vi "Overshoot Function (SubVI).vi"(0 "Signals IN":T2={"Dispense"=FALSE, "Fill"=FALSE, "Spray"=FALSE, "Drain"=TRUE, "Complete"=FALSE, "Fill Error"=FALSE, "Dispense Error"=FALSE, "Fill Timeout"=FALSE, "Dispense Timeout"=FALSE}, 1 "Values IN":T3 {"Drain Time (s)" format="%.2f"; "Drain Rate (g/sec)" format="%.2f"; "Time Elapsed (s)" format="%.2f"; "Time Target (s)" format="%.2f"; "Dynamic Setpoint (g)" format="%.2f"; "Static Setpoint (g)" format="%.2f"; "Grams to Setpoint" format="%.2f"; "Adjusted Mass (g)" format="%.2f"; "Dispense Rate (g/sec)" format="%.2f"; "Fill Mass (g)" format="%.2f"; "Fill Rate (g/sec)" format="%.2f"}, 3 "Settings":T1={"ON Settings"={"Enable Dynamic Setpoint?"=TRUE, "Enable Dynamic Dispense Time?"=TRUE, "Enable Drain Rate Functions"=TRUE, "Dispense Sample Time (s)"=0.5, "Dispense Slope Ave"=0, "ON Timeout (sec)"=600.0, "1st Setpoint (% of Target)"=0.0, "2nd Setpoint (% of Target)"=0.0, "3rd Setpoint (% of Target)"=0.0, "Measure Dispense Delay (sec)"=0.0, "Settle Slope Sample Time (s)"=0.0}, "OFF Settings"={"Drain Sample Time (s)"=0.5, "Drain Rate Ave Size"=5, "Drain Rate Limits (± g/sec)"=10.0, "Level Slope Range (± g/sec)"=0.25, "OFF Timeout (sec)"=0.0, "Near SP Slope Level (± g/sec)"=0.01, "Near Setpoint Threshold (%)"=95.0}, "Overshoot Settings"={"Time Limit (s)"=60.0, "Container MAX (g)"=1500.0, "Max FILL Slope (+/- g/sec)"=10.0, "% Overshot to Enable (>)"=0.25}, "FILL Timeout (s)"=300.0, "Full Settle Time (s)"=3.0, "Pre-Hydrate \nSpray Time (s)"=10.0, "Pre-Hydrate \nWait Time (s)"=30.0}, 5 "Measured Mass (g)":dbl) -> (14 "Signals OUT":T2={"Dispense"=FALSE, "Fill"=FALSE, "Spray"=FALSE, "Drain"=TRUE, "Complete"=FALSE, "Fill Error"=FALSE, "Dispense Error"=FALSE, "Fill Timeout"=FALSE, "Dispense Timeout"=FALSE}, 15 "Values OUT":T3 {"Drain Time (s)" format="%.2f"; "Drain Rate (g/sec)" format="%.2f"; "Time Elapsed (s)" format="%.2f"; "Time Target (s)" format="%.2f"; "Dynamic Setpoint (g)" format="%.2f"; "Static Setpoint (g)" format="%.2f"; "Grams to Setpoint" format="%.2f"; "Adjusted Mass (g)" format="%.2f"; "Dispense Rate (g/sec)" format="%.2f"; "Fill Mass (g)" format="%.2f"; "Fill Rate (g/sec)" format="%.2f"}, 17 "Fill Target (g)":dbl, 18 "Fill Time Target (s)":dbl, 19 "Complete":bool)   [LabVIEW 2009]
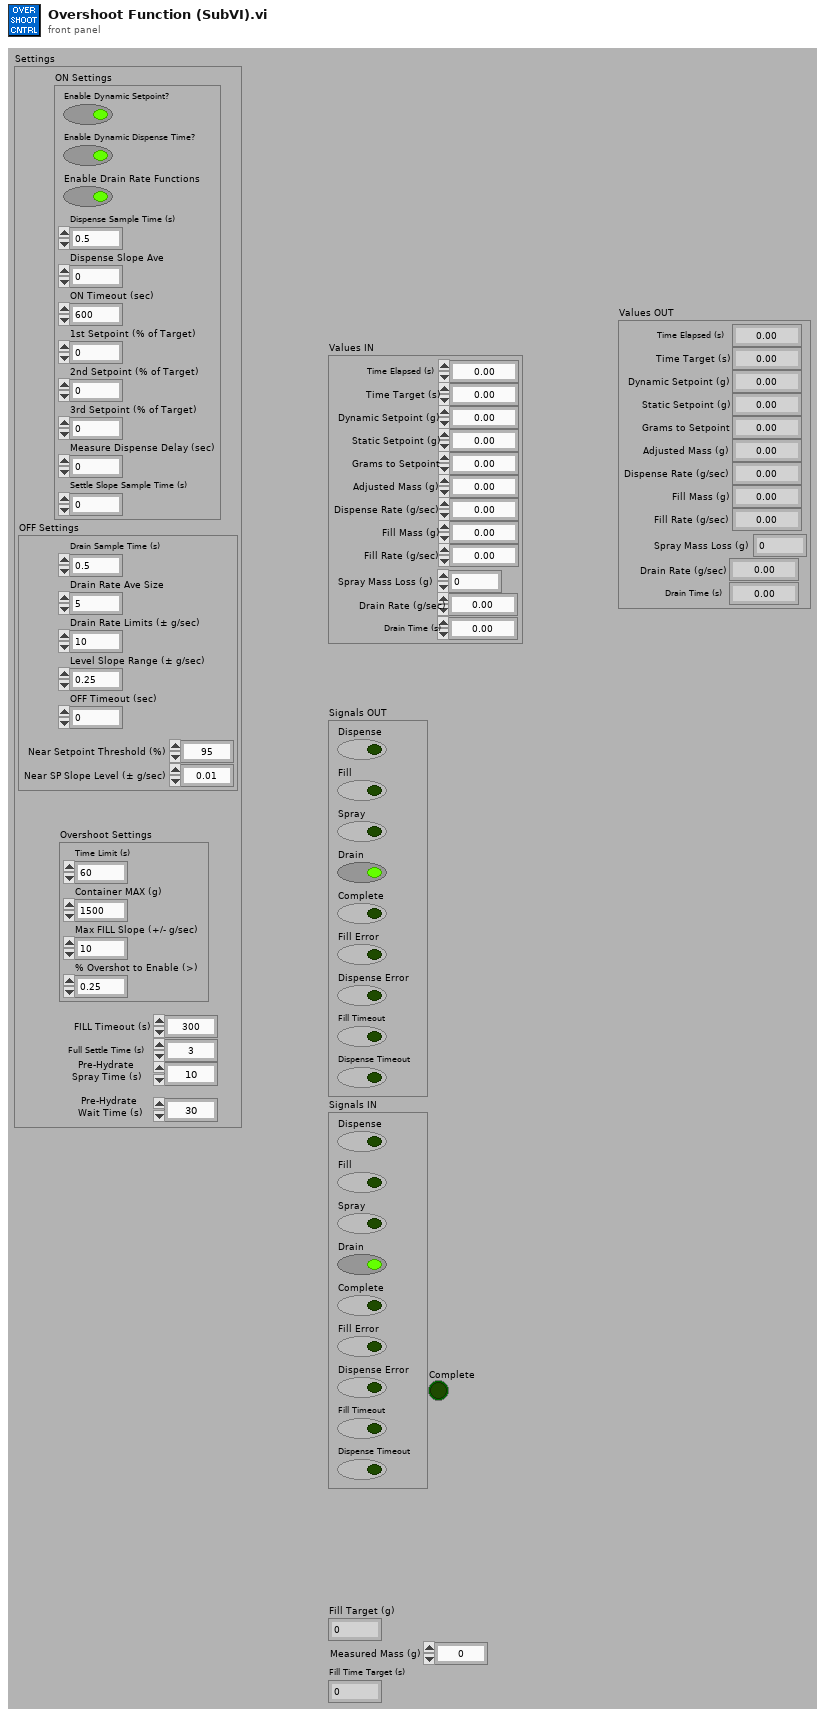
[diagram p1: front panel]
types:
  T1 = cluster{"ON Settings":cluster{"Enable Dynamic Setpoint?":bool, "Enable Dynamic Dispense Time?":bool, "Enable Drain Rate Functions":bool, "Dispense Sample Time (s)":dbl, "Dispense Slope Ave":i32, "ON Timeout (sec)":dbl, "1st Setpoint (% of Target)":dbl, "2nd Setpoint (% of Target)":dbl, "3rd Setpoint (% of Target)":dbl, "Measure Dispense Delay (sec)":dbl, "Settle Slope Sample Time (s)":dbl}, "OFF Settings":cluster{"Drain Sample Time (s)":dbl, "Drain Rate Ave Size":i32, "Drain Rate Limits (± g/sec)":dbl, "Level Slope Range (± g/sec)":dbl, "OFF Timeout (sec)":dbl, "Near SP Slope Level (± g/sec)":dbl, "Near Setpoint Threshold (%)":dbl}, "Overshoot Settings":cluster{"Time Limit (s)":dbl, "Container MAX (g)":dbl, "Max FILL Slope (+/- g/sec)":dbl, "% Overshot to Enable (>)":dbl}, "FILL Timeout (s)":dbl, "Full Settle Time (s)":dbl, "Pre-Hydrate \nSpray Time (s)":dbl, "Pre-Hydrate \nWait Time (s)":dbl}
  T2 = cluster{"Dispense":bool, "Fill":bool, "Spray":bool, "Drain":bool, "Complete":bool, "Fill Error":bool, "Dispense Error":bool, "Fill Timeout":bool, "Dispense Timeout":bool}
  T3 = cluster{"Time Elapsed (s)":dbl, "Time Target (s)":dbl, "Dynamic Setpoint (g)":dbl, "Static Setpoint (g)":dbl, "Grams to Setpoint":dbl, "Adjusted Mass (g)":dbl, "Dispense Rate (g/sec)":dbl, "Fill Mass (g)":dbl, "Fill Rate (g/sec)":dbl, "Spray Mass Loss (g)":dbl, "Drain Rate (g/sec)":dbl, "Drain Time (s)":dbl}
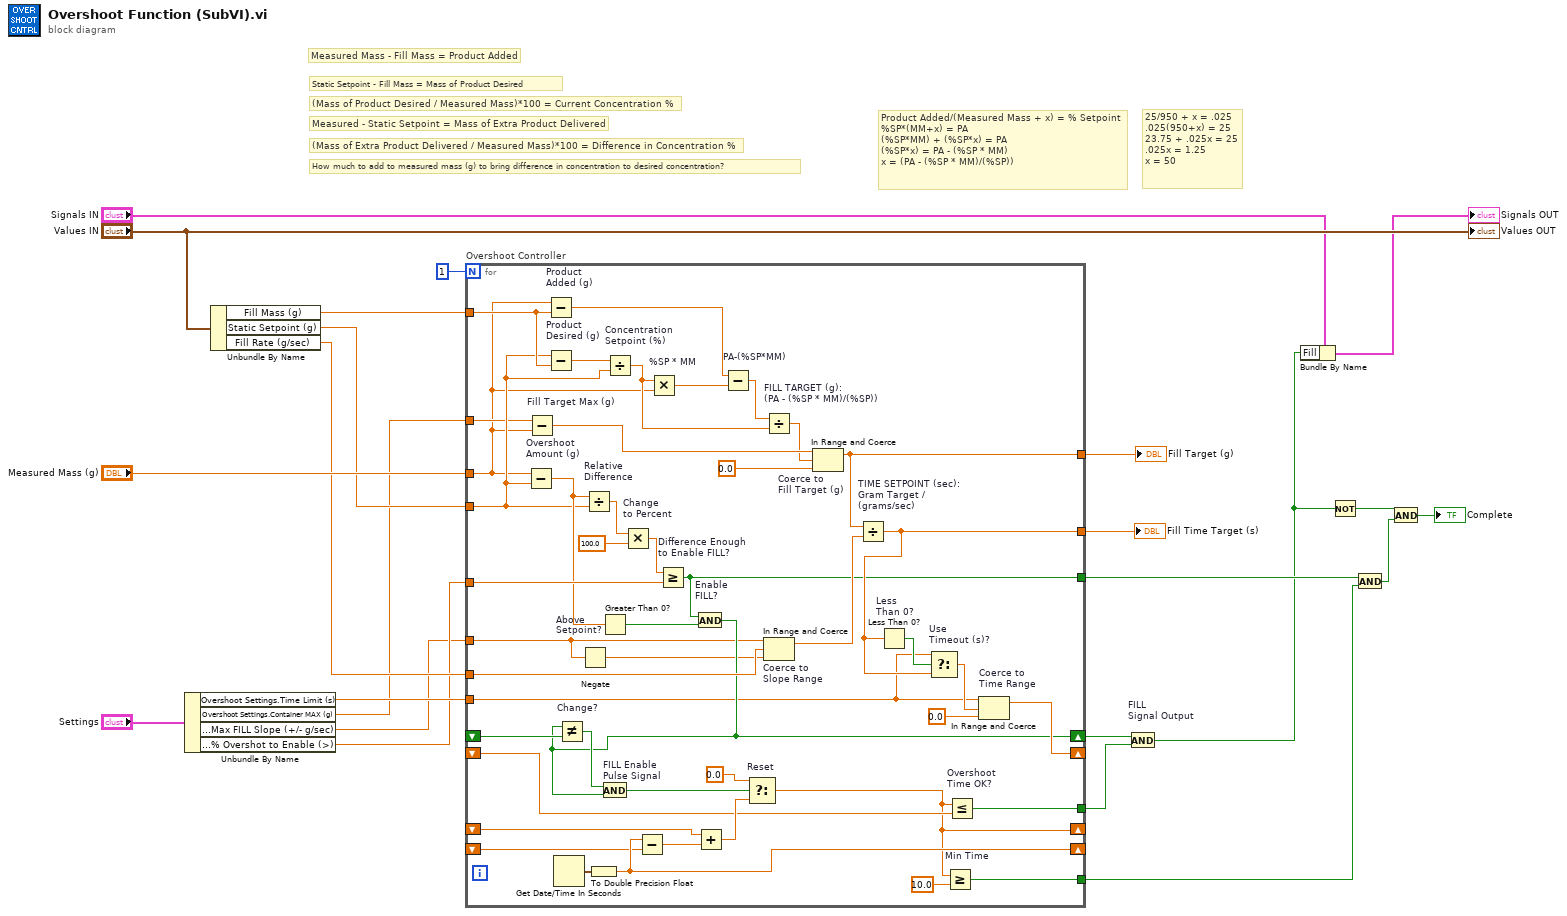
[diagram p0: block diagram]
diagram:
  # "Measured Mass - Fill Mass = Product Added"
  # "Product Added/(Measured Mass + x) = % Setpoint\n%SP*(MM+x) = PA\n(%SP*MM) + (%SP*x) = PA\n(%SP*x) = PA - (%SP * MM)\nx = (PA - (%SP * MM)/(%SP))"
  # "25/950 + x = .025\n.025(950+x) = 25\n23.75 + .025x = 25\n.025x = 1.25\nx = 50"
  # "How much to add to measured mass (g) to bring difference in concentration to desired concentration?"
  # "(Mass of Extra Product Delivered / Measured Mass)*100 = Difference in Concentration %"
  # "(Mass of Product Desired / Measured Mass)*100 = Current Concentration %"
  # "Measured - Static Setpoint = Mass of Extra Product Delivered"
  # "Static Setpoint - Fill Mass = Mass of Product Desired"
  n1 = Unbundle By Name("Settings") -> ("Overshoot Settings.Time Limit (s)"=w4:dbl, "Overshoot Settings.Container MAX (g)"=w2:dbl, "Overshoot Settings.Max FILL Slope (+/- g/sec)"=w1:dbl, "Overshoot Settings.% Overshot to Enable (>)"=w3:dbl)
  n2 = Unbundle By Name("Values IN") -> ("Fill Mass (g)"=w15:dbl, "Static Setpoint (g)"=w16:dbl, "Fill Rate (g/sec)"=w17:dbl)
  n3 = for "Overshoot Controller" {
    N: 1 -> [_]
    shift-right: [w26] -> _
    shift-left: _ -> [w69]
    shift-right: [w65] -> _
    shift-left: _ -> [w64]
    tunnel: [w66] -> w19
    shift-right: [w31] -> w20
    shift-left: _ -> [w62]
    shift-right: [w59] -> _
    shift-left: _ -> [w58]
    tunnel: w1 -> [w30]
    tunnel: w17 -> [w48]
    tunnel: w3 -> [w47]
    tunnel: w16 -> [w43]
    tunnel: "Measured Mass (g)" -> [w36]
    tunnel: w15 -> [w45]
    tunnel: [w33] -> w22
    tunnel: w2 -> [w37]
    tunnel: [w32] -> w23
    tunnel: w4 -> [w28]
    tunnel: [w27] -> w11
    tunnel: [w24] -> w10
    n4 = Subtract "Overshoot\nAmount (g)"(x=w36, y=w43) -> (x-y=w46:dbl)
    n5 = Subtract "Fill Target Max (g)"(x=w37, y=w36) -> (x-y=w35:dbl)
    n6 = Subtract "Product\nAdded (g)"(x=w36, y=w45) -> (x-y=w42:dbl)
    n7 = Subtract "Product\nDesired (g)"(x=w43, y=w45) -> (x-y=w44:dbl)
    n8 = Get Date/Time In Seconds() -> (seconds since 1Jan1904=w68:timestamp)
    n9 = Negate(x=w30) -> (-x=w29:dbl)
    n10 = Divide "Relative\nDifference"(x=w46, y=w43) -> (x/y=w50:dbl)
    n11 = To Double Precision Float(number=w68) -> (double precision float=w65:dbl)
    n12 = Greater Than 0? "Above\nSetpoint?"(x=w46) -> (x > 0?=w49:bool)
    n13 = Divide "Concentration\nSetpoint (%)"(x=w44, y=w43) -> (x/y=w39:dbl)
    n14 = Multiply "Change\nto Percent"(x=w50, y=100.0) -> (x*y=w52:dbl)
    n15 = Subtract(x=w65, y=w64) -> (x-y=w63:dbl)
    n16 = Multiply "%SP * MM"(x=w39, y=w36) -> (x*y=w41:dbl)
    n17 = Greater Or Equal? "Difference Enough\nto Enable FILL?"(x=w52, y=w47) -> (x >= y?=w27:bool)
    n18 = And "Enable\nFILL?"(x=w27, y=w49) -> (x .and. y?=w31:bool)
    n19 = Not Equal? "Change?"(x=w31, y=w62) -> (x != y?=w61:bool)
    n20 = And "FILL Enable \nPulse Signal"(x=w61, y=w31) -> (x .and. y?=w60:bool)
    n21 = Add(x=w69, y=w63) -> (x+y=w67:dbl)
    n22 = Subtract "PA-(%SP*MM)"(x=w42, y=w41) -> (x-y=w40:dbl)
    n23 = Select "Reset"(t=0.0, s=w60, f=w67) -> (s? t:f=w26:dbl)
    n24 = Divide "FILL TARGET (g):\n(PA - (%SP * MM)/(%SP))"(x=w40, y=w39) -> (x/y=w34:dbl)
    n25 = In Range and Coerce "Coerce to\nSlope Range"(upper limit=w30, x=w48, lower limit=w29) -> (coerced(x)=w53:dbl)  [unwired: 1 out]
    n26 = In Range and Coerce "Coerce to\nFill Target (g)"(upper limit=w35, x=w34, lower limit=0.0) -> (coerced(x)=w32:dbl)  [unwired: 1 out]
    n27 = Divide "TIME SETPOINT (sec):\nGram Target /\n(grams/sec)"(x=w32, y=w53) -> (x/y=w33:dbl)
    n28 = Less Than 0? "Less \nThan 0?"(x=w33) -> (x < 0?=w55:bool)
    n29 = Select "Use\nTimeout (s)?"(t=w28, s=w55, f=w33) -> (s? t:f=w54:dbl)
    n30 = Greater Or Equal? "Min Time"(x=w26, y=10.0) -> (x >= y?=w24:bool)
    n31 = Less Or Equal? "Overshoot\nTime OK?"(x=w26, y=w58) -> (x <= y?=w66:bool)
    n32 = In Range and Coerce "Coerce to\nTime Range"(upper limit=w28, x=w54, lower limit=0.0) -> (coerced(x)=w59:dbl)  [unwired: 1 out]
  }
  "Fill Time Target (s)" <- w22
  "Fill Target (g)" <- w23
  n33 = And "FILL\nSignal Output"(x=w20, y=w19) -> (x .and. y?=w9:bool)
  n34 = Bundle By Name(cluster="Signals IN", "Fill"=w9) -> (→"Signals OUT":T2)
  n35 = Not(x=w9) -> (.not. x?=w8:bool)
  n36 = And(x=w11, y=w10) -> (x .and. y?=w7:bool)
  n37 = And(x=w8, y=w7) -> (x .and. y?=→"Complete":bool)
  "Values OUT" <- "Values IN"
